vi "TimeInfoOPEN_old.vi"(7 "error in (no error)":errorcluster, 9 "Minor Time":u32, 10 "Major Time":u32) -> (0 "Date":cluster{"Date":string, "Error":string}, 1 "Open":cluster{"Time":string, "Error":string})   [LabVIEW 2015]
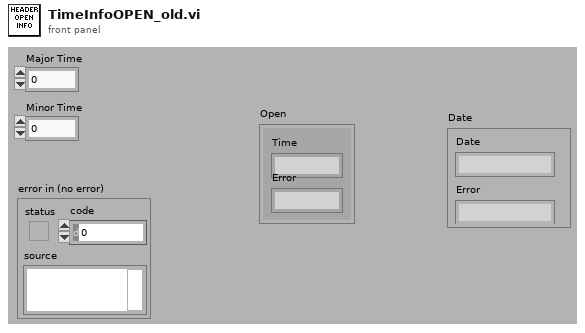
[diagram p1: front panel]
types:
  T1 = cluster{"  Open Time":string, "Open Error":string}
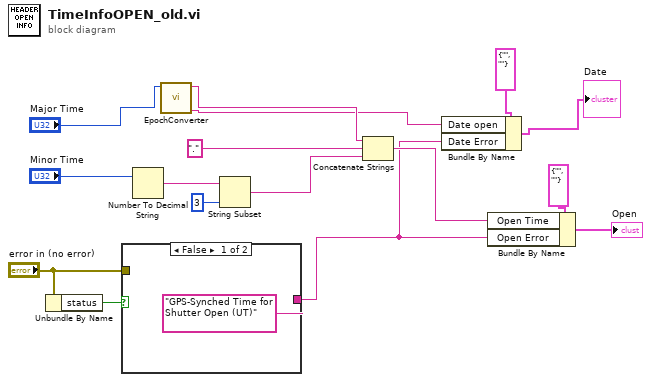
[diagram p0: block diagram]
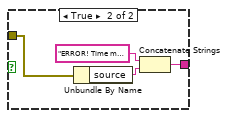
[diagram p2: hidden frame]
diagram:
  n1 = Unbundle By Name("error in (no error)") -> ("status"=w14:bool)
  n2 = case shown="False" w14 {
    tunnel: "error in (no error)" -> [_ w21]
    tunnel: ["GPS-Synched Time for Shutter Open (UT)" w20] -> w2
    frame False {
    }
    frame True {
      n3 = Unbundle By Name(w21) -> ("source"=w19:string)
      n4 = Concatenate Strings("ERROR! Time may be Invalid.  Source: ", w19) -> (w20:string)
    }
  }
  n5 = Number To Decimal String(number="Minor Time") -> (decimal integer string=w8:string)  [unwired: 1 in]
  n6 = call "EpochConverter.vi"("Epoch time"="Major Time") -> ("Date"=w4:string, "String"=w5:string)  [unwired: 9 in]
  n7 = String Subset(string=w8, length (rest)=3) -> (substring=w7:string)  [unwired: 1 in]
  n8 = Concatenate Strings(w5, ".", w7) -> (w11:string)
  n9 = Bundle By Name(cluster=cluster{"Date open":string, "Date Error":string} {"Date open"="", "Date Error"=""}, "Date open"=w4, "Date Error"=w2) -> (→"Date":cluster{"Date open":string, "Date Error":string})
  n10 = Bundle By Name(cluster=T1 {"  Open Time"="", "Open Error"=""}, "Open Time"=w11, "Open Error"=w2) -> (→"Open":T1)
